vi "Position Next Key.vi"(8 "error in (no error)":errorcluster, 10 "Previous Key":refnum<vi>, 11 "Input Key":refnum<vi>) -> (0 "error out":errorcluster)   [LabVIEW 2014]
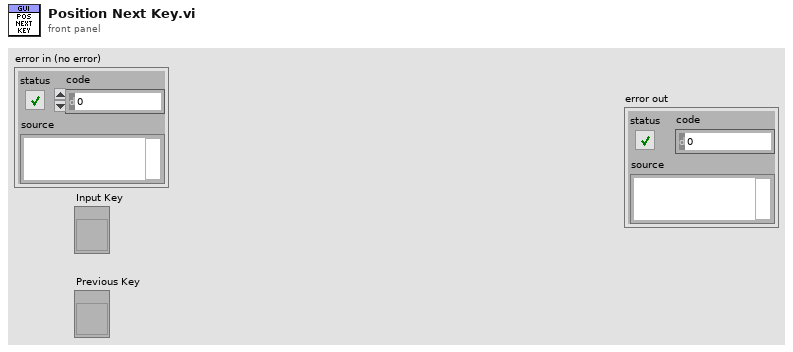
[diagram p1: front panel]
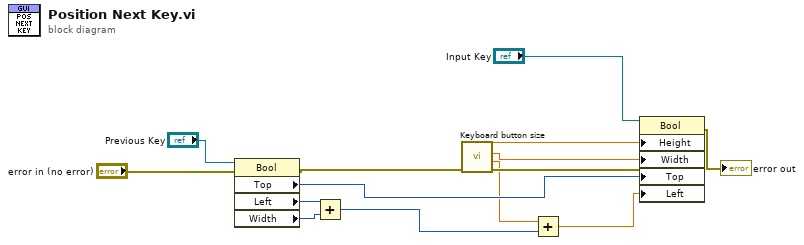
[diagram p0: block diagram]
diagram:
  n1 = property class="Bool"(reference="Previous Key", error in="error in (no error)") -> (error out=w9:errorcluster, "Top"=w6:i32, "Left"=w5:i32, "Width"=w4:u32)  [unwired: 1 out]
  n2 = Add(x=w5, y=w4) -> (x+y=w2:u32)
  n3 = call "Keyboard button size.vi"("error in (no error)"=w9) -> ("error out"=w13:errorcluster, "Key Spacing"=w3:dbl, "Key Width"=w11:dbl, "Key Height"=w10:dbl)  [unwired: 7 in]
  n4 = Add(x=w3, y=w2) -> (x+y=w1:dbl)
  n5 = property class="Bool"(reference="Input Key", error in=w13, "Height"=w10, "Width"=w11, "Top"=w6, "Left"=w1) -> (error out=→"error out":errorcluster)  [unwired: 1 out]
